vi "collect pulses.vi"(8 "error in (no error)":errorcluster, 9 "max number of pulses to show":dbl, 10 "time range":cluster{dbl, dbl}(slide)={9.216589861751153, 78525345.62211981} scale=0.0..50.0 scale format="%#_6p sec", 11 "device_type in":refnum<class "device_type.lvclass">) -> (0 "error out":errorcluster, 2 "PDW":cluster{"PDW":T1[], "Ton":dbl[]} {"PDW"."frequency shift" format="%#_12f"}, 3 "device_type out":refnum<class "device_type.lvclass">)   [LabVIEW 2021, in "device_type.lvclass"]
uses:
  device_type.lvclass
  pulse_tx_vis/pdw.ctl
  pulse_tx_vis/mode_type.ctl
  device_type.lvclass/device_type.ctl
  <vilib>/Analysis/1siggen.llb/Ramp Pattern by Delta.vi
  <instrlib>/_niInstr/Basic Elements/v1/FPGA/Private/Count Up U64.vi
  <vilib>/Analysis/NI_AALBase.lvlib
  <instrlib>/_niInstr/Basic Elements/v1/FPGA/niInstr Basic Elements v1 FPGA.lvlib
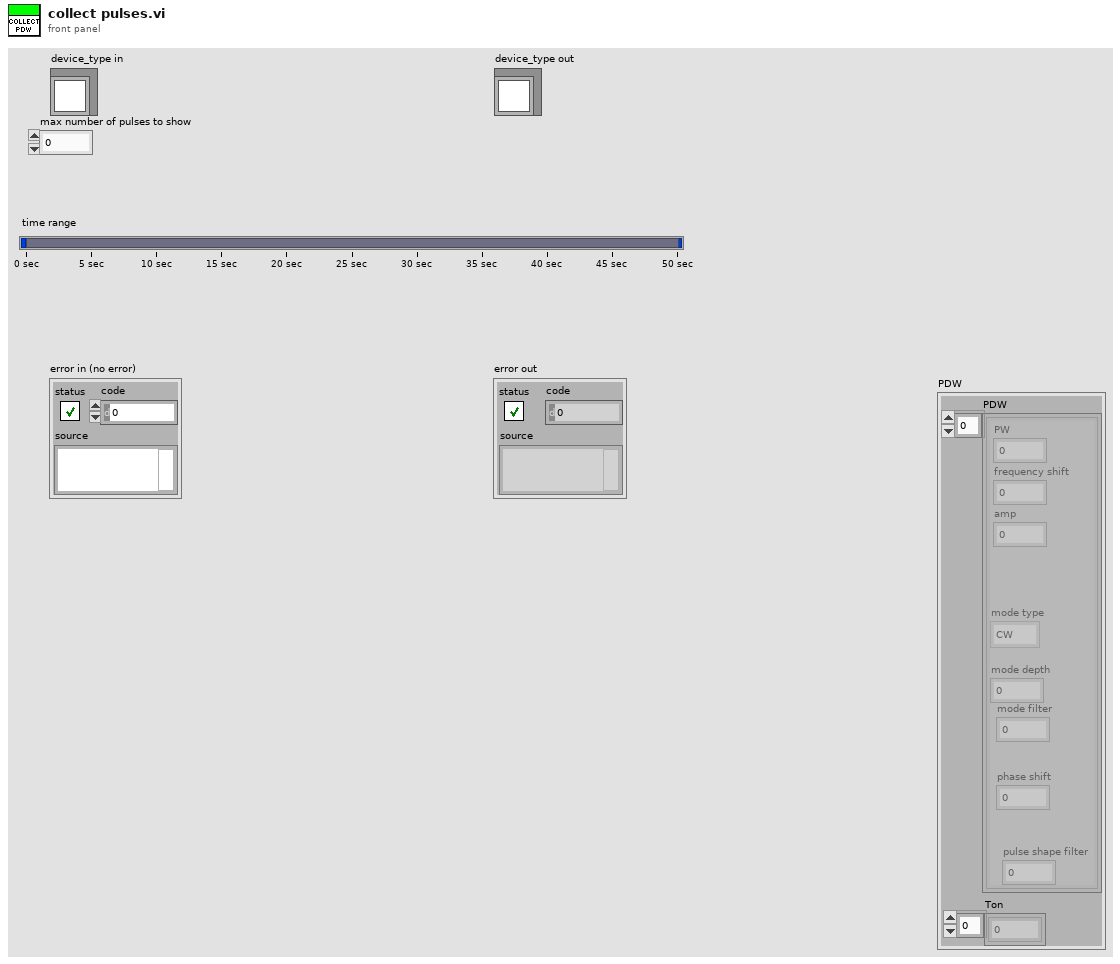
[diagram p1: front panel]
types:
  T1 = typedef "pdw.ctl" = cluster{"PW":u32, "frequency shift":fxp<+/-,48,0>, "amp":fxp<+/-,18,1>, "mode type":T2, "mode depth":u32, "mode filter":u8, "phase shift":fxp<+/-,16,1>, "pulse shape filter":u8}
  T2 = typedef "mode_type.ctl" = enum8{"CW", "NC - CW", "NC - cw", "LFM", "BPSK", "QPSK"}
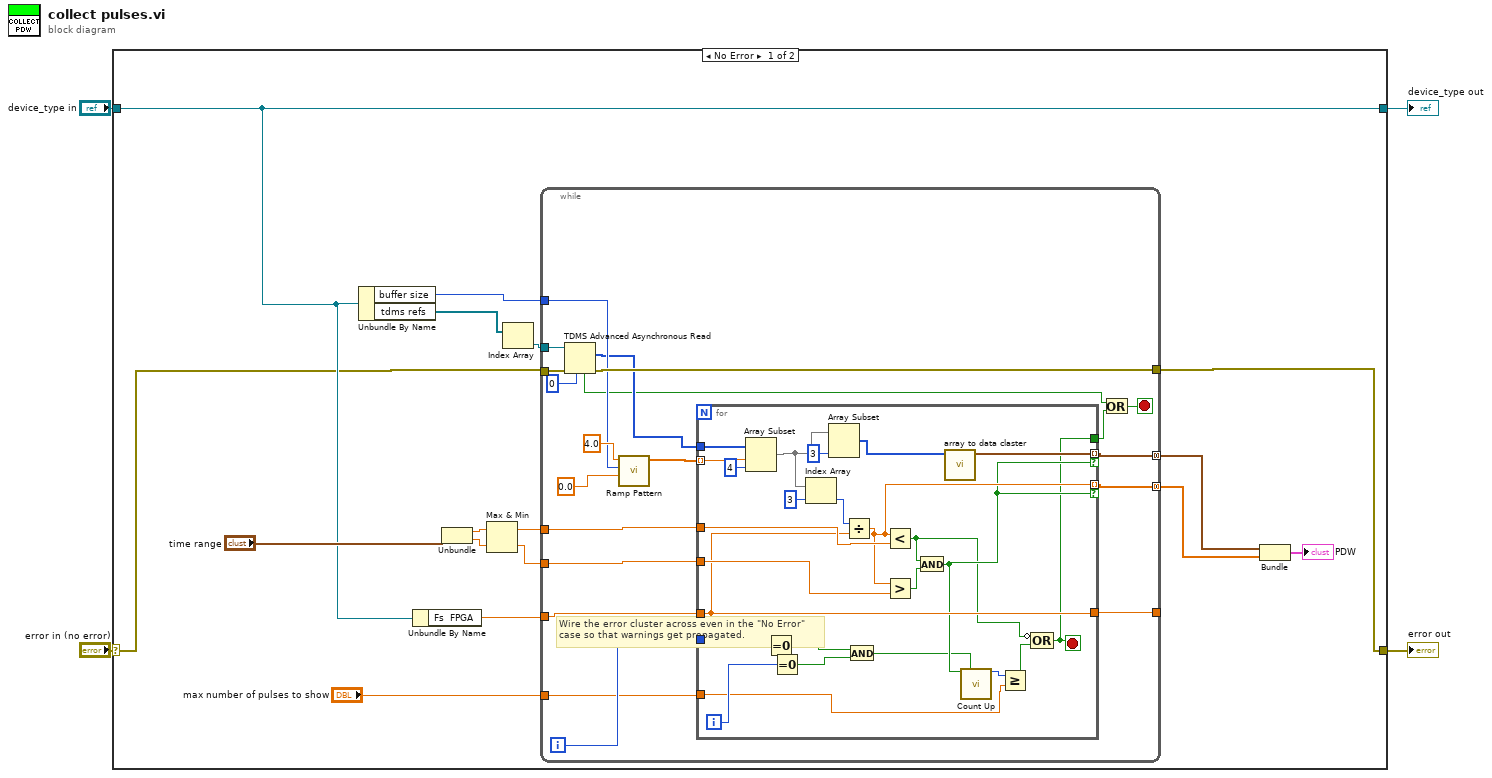
[diagram p0: block diagram]
diagram:
  n1 = case shown="No Error" "error in (no error)" {
    selector: "error in (no error)" -> [w6 w67]
    tunnel: [w5 w67] -> w3
    tunnel: [w7 w66] -> w1
    tunnel: "device_type in" -> [w7 w66]
    frame No Error {
      # "Wire the error cluster across even in the \"No Error\"\ncase so that warnings get propagated."
      n2 = Unbundle By Name(w7) -> ("buffer size"=w17:u32, "tdms refs"=w19:refnum<k34>[])
      n3 = Unbundle By Name(w7) -> ("Fs  FPGA"=w16:dbl)
      n4 = Unbundle("time range") -> (w11:dbl, w12:dbl)
      n5 = Max & Min(x=w11, y=w12) -> (max(x,y)=w15:dbl, min(x,y)=w14:dbl)
      n6 = Index Array(array=w19) -> (element=w18:refnum<k34>)  [unwired: 1 in]
      n7 = while {
        tunnel: w18 -> [w27]
        tunnel: w6 -> [w40]
        tunnel: [w39] -> w5
        tunnel: w17 -> [w36]
        tunnel: w16 -> [w33]
        tunnel: w14 -> [w32]
        tunnel: w15 -> [w31]
        tunnel: [w30] -> w9 mode=concatenating
        tunnel: [w29] -> w10 mode=concatenating
        tunnel: [w28] -> _
        tunnel: "max number of pulses to show" -> [w21]
        i -> [w25]
        stop <- w22 stop-if-true
        n8 = TDMS Advanced Asynchronous Read(6:u64 0 ("data type"), 8:w40, 11:w27) -> (0:w39:errorcluster, 2:w34:u64[], 4:w24:bool)  [unwired: 1 out]
        n9 = call-poly <vilib>:"Ramp Pattern.vi"("start"=0.0, "end"=w36, "delta"=4.0) -> ("Ramp Pattern"=w35:dbl[])  [unwired: 6 in, 2 out]
        n10 = for {
          tunnel: w35 -> [w65] mode=indexing
          tunnel: w34 -> [w64]
          tunnel: w33 -> [w55]
          tunnel: w32 -> [w60]
          tunnel: w31 -> [w59]
          tunnel: [w57] -> w29 mode=indexing if=w51
          tunnel: [w56] -> w30 mode=indexing if=w51
          tunnel: [w55] -> w28
          tunnel: w25 -> [w46]
          tunnel: [w42] -> w23
          tunnel: w21 -> [w41]
          i -> [w47]
          stop <- w42 stop-if-true
          n11 = Array Subset(array=w64, index=w65, length=4) -> (w54:u64[])
          n12 = Equal To 0?(x=w46) -> (x = 0?=w45:bool)
          n13 = Equal To 0?(x=w47) -> (x = 0?=w44:bool)
          n14 = Index Array(array=w54, index=3) -> (element=w61:u64)
          n15 = Array Subset(array=w54, length=3) -> (w52:u64[])  [unwired: 1 in]
          n16 = Divide(x=w61, y=w55) -> (x/y=w56:dbl)
          n17 = And(x=w45, y=w44) -> (x .and. y?=w43:bool)
          n18 = Less?(x=w56, y=w59) -> (x < y?=w49:bool)
          n19 = Greater?(x=w56, y=w60) -> (0:w58:bool)
          n20 = And(x=w49, y=w58) -> (x .and. y?=w51:bool)
          n21 = call "array to data claster.vi"("Array"=w52) -> ("Cluster"=w57:T1)  [unwired: 10 in]
          n22 = call-poly <instrlib>:"Count Up.vi"("increment"=w51, "reset"=w43) -> ("count out"=w50:u64)  [unwired: 13 in]
          n23 = Greater Or Equal?(x=w50, y=w41) -> (x >= y?=w48:bool)
          n24 = Compound Arithmetic op=OR(invert w49, w48) -> (w42:bool)
        }
        n25 = Or(x=w24, y=w23) -> (x .or. y?=w22:bool)
      }
      n26 = Bundle(w10, w9) -> (→"PDW":cluster{T1[], dbl[]})  [unwired: 1 in]
    }
    frame Error {
    }
  }
  "error out" <- w3
  "device_type out" <- w1
